vi "PathPlanner_Path_CreatePath_Worker2.vi"(4 "GlobalConstraints":T3, 6 "ConstraintZones":T7[](array[typedef]), 7 "Waypoints":T6[](array[typedef]) {"nextControl"."Y" format="%14.3f"; "nextControl"."X" format="%14.3f"; "anchor"."Y" format="%14.3f"; "anchor"."X" format="%14.3f"; "prevControl"."Y" format="%14.3f"; "prevControl"."X" format="%14.3f"}, 8 "TrueIncrement":dbl, 9 "NumSegments":dbl, 10 "UnaddedTargets":T4[](array[typedef]) {"rotation"."SIN" format="%13.4f"; "rotation"."COS" format="%13.4f"; "rotation"."VALUE" format="%13.4f"}, 11 "Points in":T1[](array[typedef]) {"RotationTarget"."rotation"."SIN" format="%13.4f"; "RotationTarget"."rotation"."COS" format="%13.4f"; "RotationTarget"."rotation"."VALUE" format="%13.4f"; "Position"."Y" format="%14.3f"; "Position"."X" format="%14.3f"}) -> (3 "Points out":T1[](array[typedef]) {"RotationTarget"."rotation"."SIN" format="%13.4f"; "RotationTarget"."rotation"."COS" format="%13.4f"; "RotationTarget"."rotation"."VALUE" format="%13.4f"; "Position"."Y" format="%14.3f"; "Position"."X" format="%14.3f"})   [LabVIEW 2019, in "PathPlanner24.lvlib"]
doc: "Internal function for CreatePath -- DO NOT CALL."
uses:
  PathPlanner24.lvlib
  TypeDef/PathPlannerPathPoint.ctl
  <vilib>/Rock Robotics/WPI/ThirdParty/JAS_Junk/TrajLib/TypeDef/TRANSLATION2D.ctl
  TypeDef/PathPlannerPathConstraints.ctl
  TypeDef/PathPlannerRotationTarget.ctl
  <vilib>/Rock Robotics/WPI/ThirdParty/JAS_Junk/TrajLib/TypeDef/ROTATION2D.ctl
  TypeDef/PathPlannerConstraintsZone.ctl
  TypeDef/PathPlannerWaypoint.ctl
  <vilib>/Rock Robotics/WPI/ThirdParty/JAS_Junk/TrajLib/MathUtil_Clamp.vi
  <vilib>/Rock Robotics/WPI/ThirdParty/JAS_Junk/TrajLib/Util_CalcDist.vi
  PathPlanner_PathConstraints_UnlimitedConstraints.vi
  PathPlanner_GeomUtil_CubicLerp.vi
  <vilib>/Rock Robotics/WPI/ThirdParty/JAS_Junk/TrajLib/Trajectory_Library.lvlib
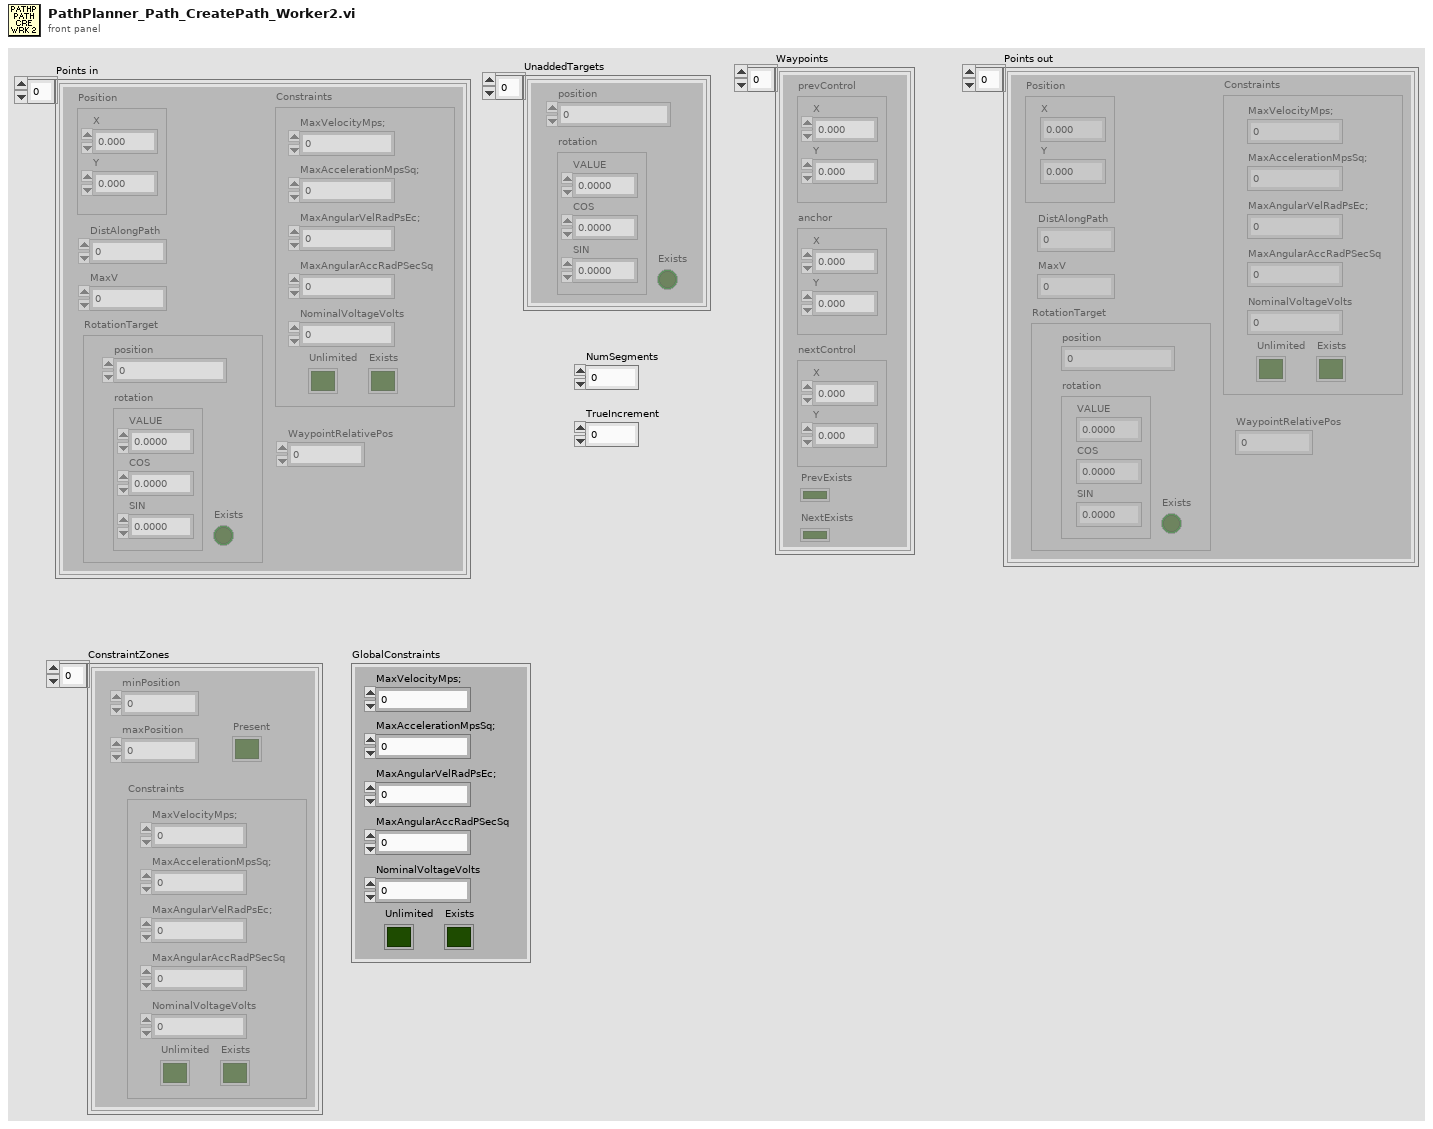
[diagram p1: front panel]
types:
  T1 = typedef "PathPlanner24.lvlib/PathPlannerPathPoint.ctl" = cluster{"Position":T2, "DistAlongPath":dbl, "MaxV":dbl, "Constraints":T3, "RotationTarget":T4, "WaypointRelativePos":dbl}
  T2 = typedef "Trajectory_Library.lvlib/TRANSLATION2D.ctl" = cluster{"X":dbl, "Y":dbl}
  T3 = typedef "PathPlanner24.lvlib/PathPlannerPathConstraints.ctl" = cluster{"MaxVelocityMps;":dbl, "MaxAccelerationMpsSq;":dbl, "MaxAngularVelRadPsEc;":dbl, "MaxAngularAccRadPSecSq":dbl, "Exists":bool, "Unlimited":bool, "NominalVoltageVolts":dbl}
  T4 = typedef "PathPlanner24.lvlib/PathPlannerRotationTarget.ctl" = cluster{"position":dbl, "rotation":T5, "Exists":bool}
  T5 = typedef "Trajectory_Library.lvlib/ROTATION2D.ctl" = cluster{"VALUE":dbl, "COS":dbl, "SIN":dbl}
  T6 = typedef "PathPlanner24.lvlib/PathPlannerWaypoint.ctl" = cluster{"prevControl":T2, "anchor":T2, "nextControl":T2, "PrevExists":bool, "NextExists":bool}
  T7 = typedef "PathPlanner24.lvlib/PathPlannerConstraintsZone.ctl" = cluster{"minPosition":dbl, "maxPosition":dbl, "Constraints":T3, "Present":bool}
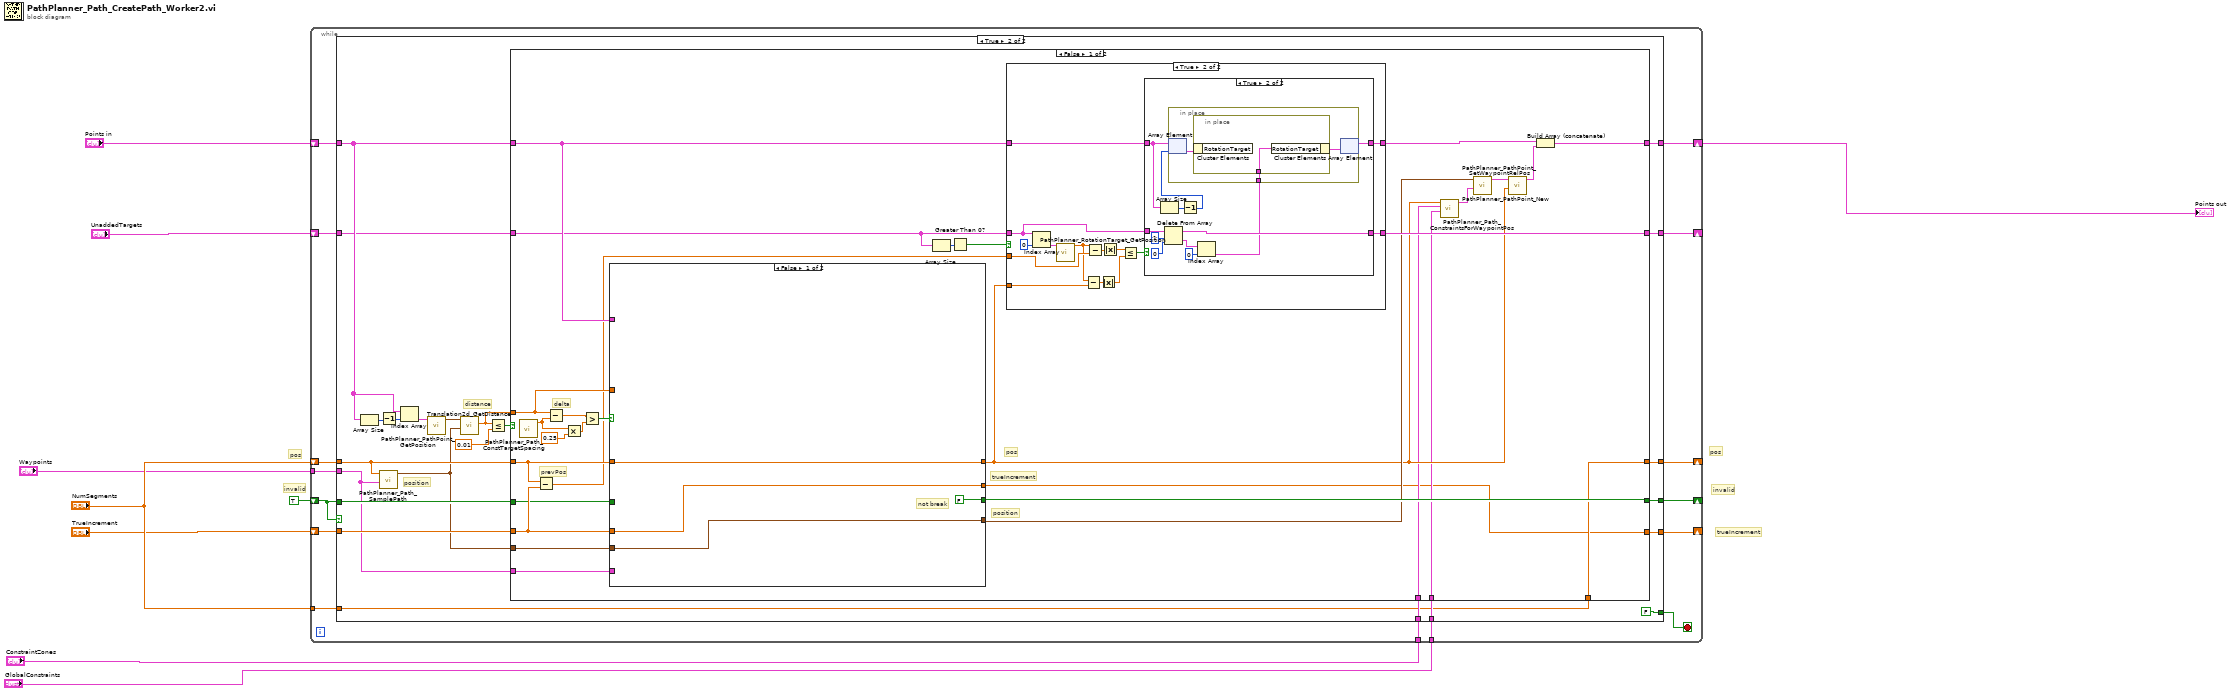
[diagram p0: block diagram]
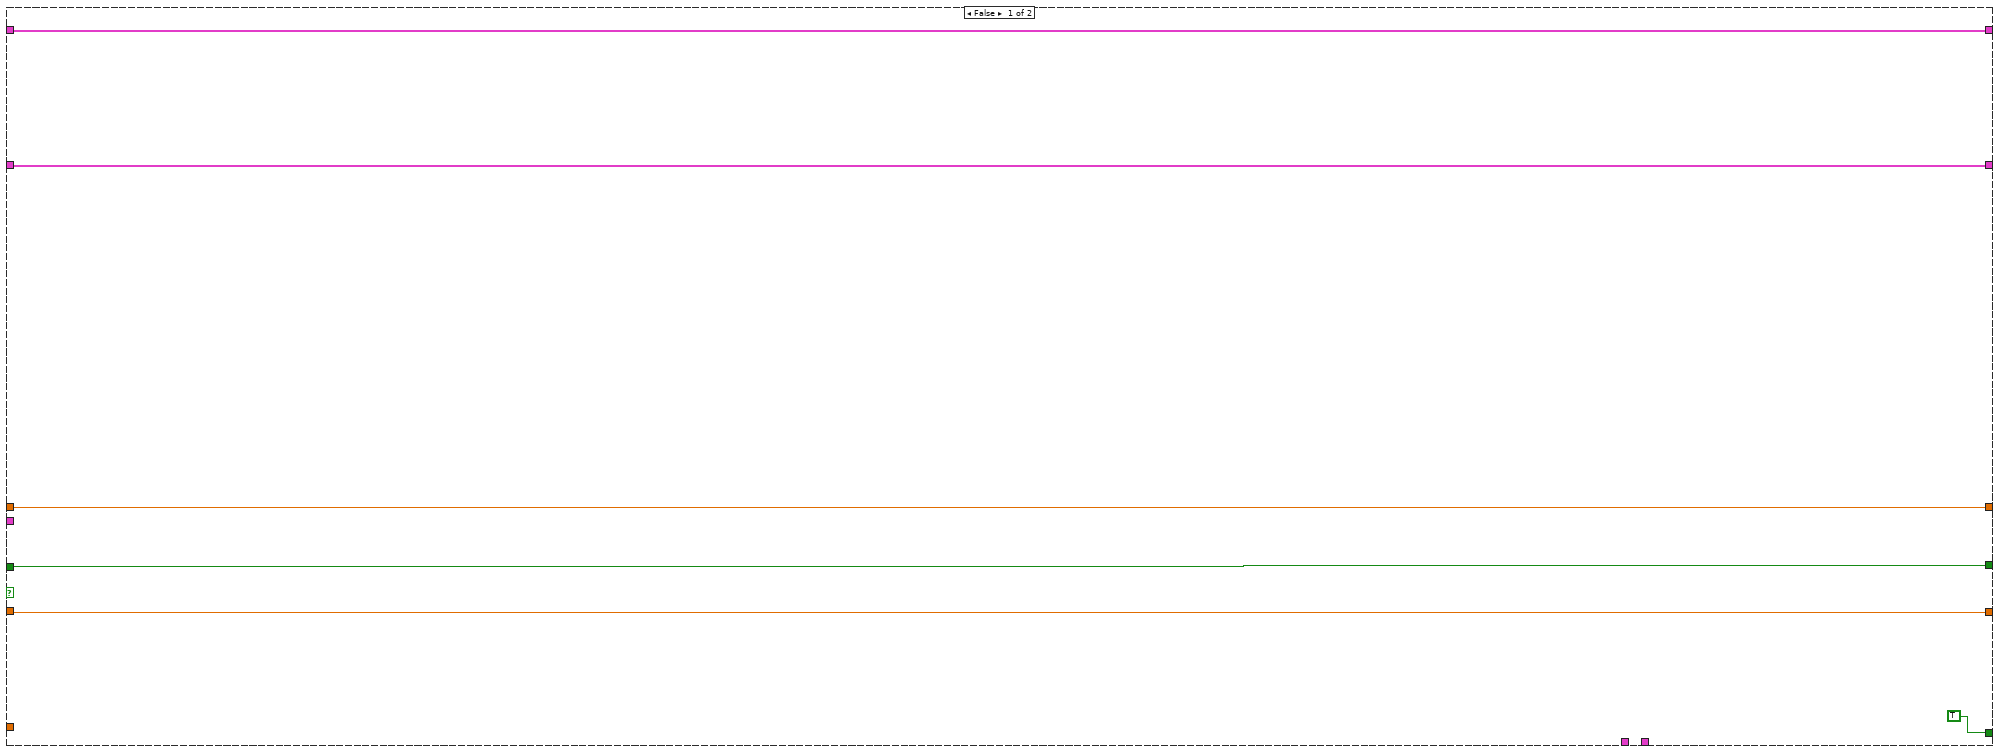
[diagram p2: hidden frame]
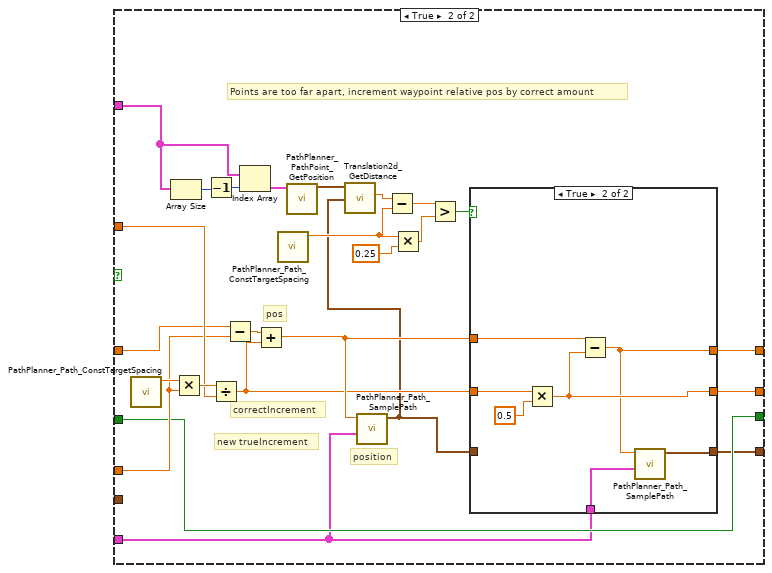
[diagram p5: hidden frame]
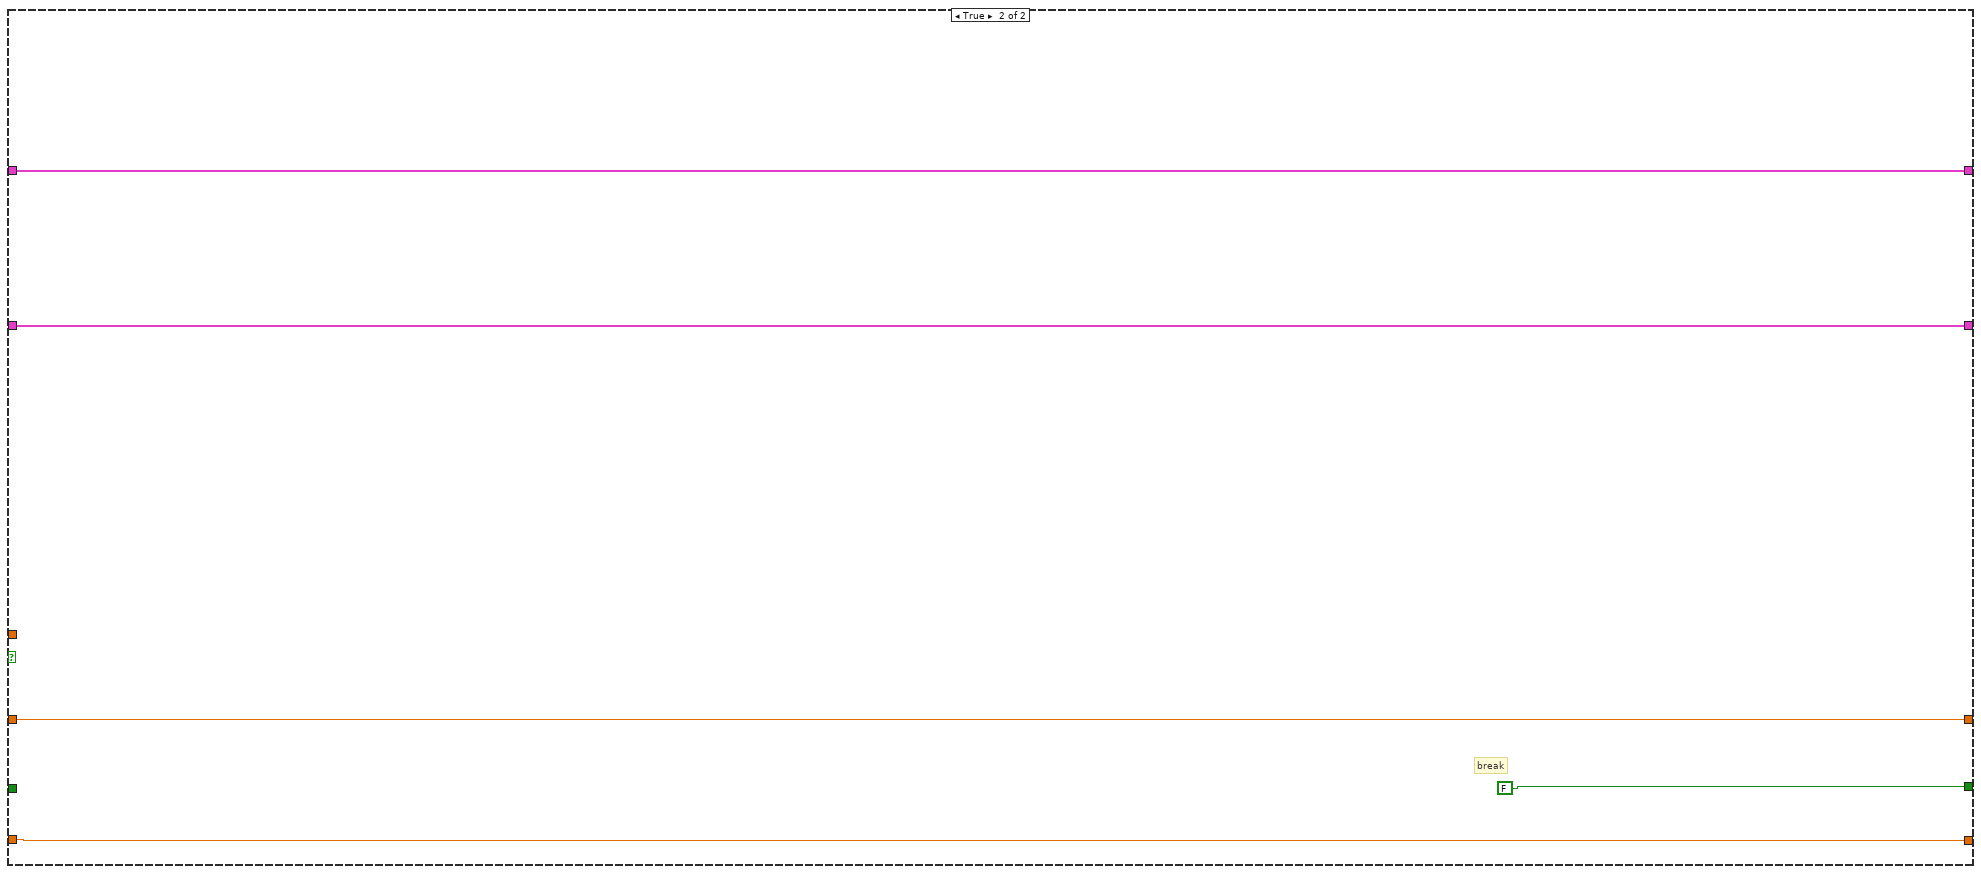
[diagram p7: hidden frame]
diagram:
  # "trueIncrement"
  # "pos"
  # "invalid"
  # "pos"
  # "invalid"
  n1 = while {
    shift-right: [w17] -> w9
    shift-left: "Points in" -> [w21]
    shift-right: [w20] -> _
    shift-left: TRUE -> [w18]
    shift-right: [w19] -> _
    shift-left: "NumSegments" -> [w23]
    tunnel: "Waypoints" -> [w22]
    shift-right: [w14] -> _
    shift-left: "UnaddedTargets" -> [w15]
    tunnel: "ConstraintZones" -> [w13]
    tunnel: "GlobalConstraints" -> [w12]
    tunnel: "NumSegments" -> [w11]
    shift-right: [w10] -> _
    shift-left: "TrueIncrement" -> [w16]
    stop <- w24 stop-if-true
    n2 = case shown="True" w18 {
      tunnel: [TRUE FALSE] -> w24
      tunnel: w23 -> [w28 w45]
      tunnel: w22 -> [_ w38]
      tunnel: w21 -> [w27 w42]
      tunnel: [w29 w47] -> w20
      tunnel: [w28 w44] -> w19
      tunnel: w18 -> [w29 w43]
      tunnel: [w27 w41] -> w17
      tunnel: w16 -> [w25 w40]
      tunnel: w15 -> [w26 w36]
      tunnel: [w26 w35] -> w14
      tunnel: w13 -> [_ w34]
      tunnel: w12 -> [_ w33]
      tunnel: w11 -> [_ w32]
      tunnel: [w25 w31] -> w10
      frame False {
      }
      frame True {
        # "distance"
        # "position"
        n3 = Array Size(array=w42) -> (size(s)=w52:i32)
        n4 = call "PathPlanner_Path_SamplePath.vi"("Waypoints"=w38, "WaypointRelativePos"=w45) -> ("Sample"=w37:T2)  [unwired: 9 in]
        n5 = Decrement(x=w52) -> (x-1=w51:i32)
        n6 = Index Array(array=w42, index=w51) -> (element=w50:T1)
        n7 = call "PathPlanner_PathPoint_GetPosition.vi"("PathPlannerPoint"=w50) -> ("Position"=w49:T2)  [unwired: 10 in]
        n8 = call <vilib>:"Translation2d_GetDistance.vi"("other Translation"=w37, "In Translation"=w49) -> ("Distance"=w39:dbl)  [unwired: 9 in]
        n9 = Less Or Equal?(x=w39, y=0.01) -> (x <= y?=w46:bool)
        n10 = case shown="False" w46 {
          tunnel: [w78 FALSE] -> w47
          tunnel: w45 -> [w76 w158]
          tunnel: [w55 w158] -> w44
          tunnel: w43 -> [w72 _]
          tunnel: w42 -> [w68 w157]
          tunnel: [w63 w157] -> w41
          tunnel: w40 -> [w75 w155]
          tunnel: w39 -> [w74 _]
          tunnel: w38 -> [w73 _]
          tunnel: w37 -> [w71 _]
          tunnel: w36 -> [w67 w156]
          tunnel: [w66 w156] -> w35
          tunnel: w34 -> [w57 _]
          tunnel: w33 -> [w56 _]
          tunnel: w32 -> [w55 _]
          tunnel: [w54 w155] -> w31
          frame False {
            # "position"
            # "trueIncrement"
            # "pos"
            # "delta"
            # "prevPos"
            n11 = call "PathPlanner_Path_ConstTargetSpacing.vi"() -> ("TargetSpacing"=w82:dbl)  [unwired: 11 in]
            n12 = Subtract(x=w76, y=w75) -> (x-y=w65:dbl)
            n13 = Subtract(x=w74, y=w82) -> (x-y=w80:dbl)
            n14 = Multiply(x=w82, y=0.25) -> (x*y=w79:dbl)
            n15 = Greater?(x=w80, y=w79) -> (0:w77:bool)
            n16 = case shown="False" w77 {
              tunnel: [FALSE w125] -> w78
              tunnel: w68 -> [_ w135]
              tunnel: w76 -> [w118 w141]
              tunnel: [w118 w127] -> w58
              tunnel: w75 -> [w117 w140]
              tunnel: w74 -> [_ w142]
              tunnel: w73 -> [_ w120]
              tunnel: w72 -> [_ w125]
              tunnel: [w117 w123] -> w54
              tunnel: [w116 w121] -> w60
              tunnel: w71 -> [w116 _]
              frame False {
                # "not break"
              }
              frame True {
                # "position"
                # "new trueIncrement"
                # "pos"
                # "correctIncrement"
                # "Points are too far apart, increment waypoint relative pos by correct amount"
                n17 = call "PathPlanner_Path_ConstTargetSpacing.vi"() -> ("TargetSpacing"=w144:dbl)  [unwired: 11 in]
                n18 = Array Size(array=w135) -> (size(s)=w138:i32)
                n19 = Multiply(x=w144, y=w140) -> (x*y=w143:dbl)
                n20 = Decrement(x=w138) -> (x-1=w137:i32)
                n21 = Divide(x=w143, y=w142) -> (x/y=w124:dbl)
                n22 = Subtract(x=w141, y=w140) -> (x-y=w139:dbl)
                n23 = Index Array(array=w135, index=w137) -> (element=w136:T1)
                n24 = Add(x=w139, y=w124) -> (x+y=w126:dbl)
                n25 = call "PathPlanner_Path_ConstTargetSpacing.vi"() -> ("TargetSpacing"=w130:dbl)  [unwired: 11 in]
                n26 = call "PathPlanner_PathPoint_GetPosition.vi"("PathPlannerPoint"=w136) -> ("Position"=w134:T2)  [unwired: 10 in]
                n27 = call "PathPlanner_Path_SamplePath.vi"("Waypoints"=w120, "WaypointRelativePos"=w126) -> ("Sample"=w122:T2)  [unwired: 9 in]
                n28 = call <vilib>:"Translation2d_GetDistance.vi"("other Translation"=w122, "In Translation"=w134) -> ("Distance"=w133:dbl)  [unwired: 9 in]
                n29 = Subtract(x=w133, y=w130) -> (x-y=w132:dbl)
                n30 = Multiply(x=w130, y=0.25) -> (x*y=w129:dbl)
                n31 = Greater?(x=w132, y=w129) -> (0:w128:bool)
                n32 = case shown="True" w128 {
                  tunnel: [w147 w148] -> w127
                  tunnel: w126 -> [w147 w152]
                  tunnel: w124 -> [w145 w153]
                  tunnel: [w145 w151] -> w123
                  tunnel: w122 -> [w146 _]
                  tunnel: [w146 w149] -> w121
                  tunnel: w120 -> [_ w150]
                  frame False {
                  }
                  frame True {
                    n33 = Multiply(x=w153, y=0.5) -> (x*y=w151:dbl)
                    n34 = Subtract(x=w152, y=w151) -> (x-y=w148:dbl)
                    n35 = call "PathPlanner_Path_SamplePath.vi"("Waypoints"=w150, "WaypointRelativePos"=w148) -> ("Sample"=w149:T2)  [unwired: 9 in]
                  }
                }
              }
            }
            n36 = Array Size(array=w67) -> (size(s)=w70:i32)
            n37 = Greater Than 0?(x=w70) -> (x > 0?=w69:bool)
            n38 = case shown="True" w69 {
              tunnel: w68 -> [w83 w86]
              tunnel: w67 -> [w84 w88]
              tunnel: [w84 w87] -> w66
              tunnel: [w83 w85] -> w64
              tunnel: w65 -> [_ w96]
              tunnel: w58 -> [_ w91]
              frame False {
              }
              frame True {
                n39 = Index Array(array=w88, index=0) -> (element=w97:T4)
                n40 = call "PathPlanner_RotationTarget_GetPosition.vi"("RotationTarget"=w97) -> ("position"=w92:dbl)  [unwired: 9 in, 1 out]
                n41 = Subtract(x=w92, y=w91) -> (x-y=w93:dbl)
                n42 = Subtract(x=w92, y=w96) -> (x-y=w95:dbl)
                n43 = Absolute Value(x=w93) -> (abs(x)=w90:dbl)
                n44 = Absolute Value(x=w95) -> (abs(x)=w94:dbl)
                n45 = Less Or Equal?(x=w94, y=w90) -> (x <= y?=w89:bool)
                n46 = case shown="True" w89 {
                  tunnel: w88 -> [w100 w111]
                  tunnel: [w100 w108] -> w87
                  tunnel: w86 -> [w99 w106]
                  tunnel: [w99 w104] -> w85
                  frame False {
                  }
                  frame True {
                    n47 = Array Size(array=w106) -> (size(s)=w107:i32)
                    n48 = Delete From Array(array=w111, length=1, index=0) -> (deleted portion=w103:T4[], array with subset deleted=w108:T4[])
                    n49 = Decrement(x=w107) -> (x-1=w105:i32)
                    n50 = Index Array(array=w103, index=0) -> (element=w101:T4)
                    n51 = in-place {
                      in-place-border: w101 -> [w112]
                      n52 = in-place-array #1(w106, w105) -> (w114:T1)
                      n53 = in-place {
                        in-place-border: w112 -> [w115]
                        n54 = in-place-cluster #2(w114) -> ()  [unwired: 1 out]
                        n55 = in-place-cluster #2("RotationTarget"=w115) -> (w113:T1)
                      }
                      n56 = in-place-array #1(w113) -> (w104:T1[])  [unwired: 1 out]
                    }
                  }
                }
              }
            }
            n57 = call "PathPlanner_Path_ConstraintsForWaypointPos.vi"("GlobalConstraints"=w56, "ConstraintsZones"=w57, "Pos"=w58) -> ("outPathPlannerPathConstraints"=w59:T3)  [unwired: 8 in]
            n58 = call "PathPlanner_PathPoint_New.vi"("Constraints"=w59, "Position"=w60) -> ("PathPlannerPoint"=w62:T1)  [unwired: 9 in]
            n59 = call "PathPlanner_PathPoint_SetWaypointRelPos.vi"("WaypointRelativePos"=w58, "PathPlannerPoint"=w62) -> ("outPathPlannerPoint"=w61:T1)  [unwired: 9 in]
            n60 = Build Array (concatenate)(w64, w61) -> (w63:T1[])
          }
          frame True {
            # "break"
          }
        }
      }
    }
  }
  "Points out" <- w9
